vi "Read from Hardware.vi"(8 "error in":errorcluster, 10 "Values in":dbl[](array[numeric]), 11 "Monitor Execution Unit Implementation in":refnum<class "Monitor Execution Unit.lvclass">) -> (0 "error out":errorcluster, 2 "Values out":dbl[](array[numeric]), 3 "Monitor Execution Unit Implementation out":refnum<class "Monitor Execution Unit.lvclass">)   [LabVIEW 2020, in "AIM ARINC 664 Engine.lvlib" / "Implementation.lvlib" / "Monitor Execution Unit.lvclass"]
uses:
  Monitor Execution Unit.lvclass
  Monitor Execution Unit.lvclass/Monitor Execution Unit.ctl
  <instrlib>/AIM GmbH/_AIM 664/AIM664LV.lvlib
  Logging/Frame Logging/Frame Logging.lvlib
  <vilib>/Utility/SystemLogging/NI_SystemLogging.lvlib
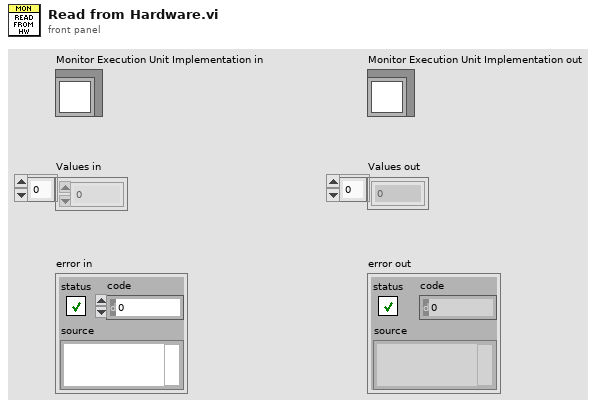
[diagram p1: front panel]
types:
  T1 = typedef "Frame Logging.lvlib/Log_Producer.ctl" = cluster{"Configured":bool, "message queue in":refnum<queue>, "StopNotification":refnum<notifier>}
  T2 = cluster{"QueueStatus":u32, "FramesToRead":u32, "BytesToRead":u32}
  T3 = cluster{"EntryRead":u32, "BytesRead":u32, "Synchronized":u32, "ReadBuffer":u8[]}
  T4 = typedef "Frame.ctl" = cluster{"FwIrigTime":cluster{"TtHigh":u32, "TtLow":u32}, "Payload":u8[], "Lenght":u32}
  T5 = cluster{"TotalByteCount":u32[], "FrameGoodCount":u32[], "FrameErrorCount":u32[], "BytesPerSecond":u32[], "FramesPerSecond":u32[], "PhysErrorCount":u32[], "PreamErrorCount":u32[], "UnaligErrorCount":u32[], "CRCErrorCount":u32[], "IFGErrorCount":u32[], "IPErrorCount":u32[], "MACErrorCount":u32[], "NoSfdErrorCount":u32[], "VLLenErrorCount":u32[], "SNIntegrityErrorCount":u32[], "TrafShapingViolationCount":u32[], "MAC1Short":u32[], "MAC64To127Count":u32[], "MAC128To255Count":u32[], "MAC256To511Count":u32[], "MAC512To1023Count":u32[], "MAC1024To1518Count":u32[], "MACLong":u32[]}
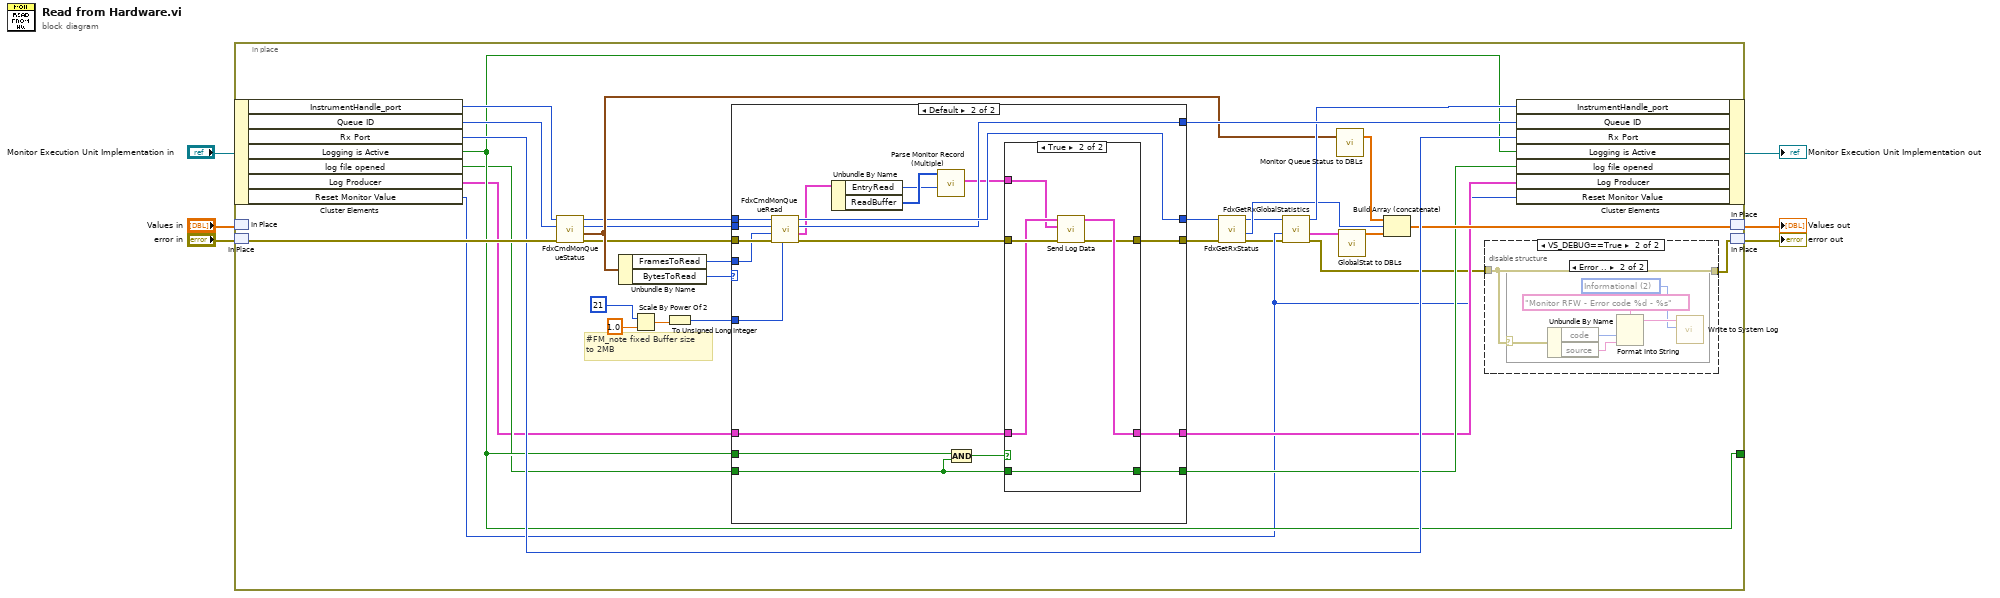
[diagram p0: block diagram]
diagram:
  n1 = in-place {
    in-place-border: [w29] -> _
    # "#FM_note fixed Buffer size\nto 2MB"
    n2 = in-place-cluster #1("Monitor Execution Unit Implementation in") -> ("InstrumentHandle_port"=w38:u32, "Queue ID"=w39:u32, "Rx Port"=w31:u32, "Logging is Active"=w29:bool, "log file opened"=w28:bool, "Log Producer"=w26:T1, "Reset Monitor Value"=w18:u32)
    n3 = in-place-match #2("Values in") -> ()  [unwired: 1 out]
    n4 = in-place-match #3("error in") -> (w37:errorcluster)
    n5 = call <instrlib>:"FdxCmdMonQueueStatus.vi"("error in"=w37, "QueueId"=w39, "InstrumentHandle_port"=w38) -> ("error out"=w24:errorcluster, "QueueStatus"=w32:T2, "QueueIdOut"=w22:u32, "InstrumentHandle_port"=w23:u32)  [unwired: 5 in]
    n6 = Unbundle By Name(w32) -> ("FramesToRead"=w21:u32, "BytesToRead"=w11:u32)
    n7 = Scale By Power Of 2(n=21, x=1.0) -> (x*2^n=w8:dbl)
    n8 = To Unsigned Long Integer(number=w8) -> (unsigned 32bit integer=w7:u32)
    n9 = case shown="Default" w11 {
      tunnel: w24 -> [w42 w61]
      tunnel: w23 -> [w44 w63]
      tunnel: w22 -> [w43 w62]
      tunnel: [w44 w60] -> w34
      tunnel: [w43 w59] -> w35
      tunnel: [w42 w56] -> w36
      tunnel: w21 -> [_ w58]
      tunnel: w29 -> [_ w53]
      tunnel: [w41 w54] -> w27
      tunnel: w28 -> [w41 w51]
      tunnel: w26 -> [w40 w50]
      tunnel: [w40 w49] -> w25
      tunnel: w7 -> [_ w48]
      frame 0 {
      }
      frame Default {
        n10 = call <instrlib>:"FdxCmdMonQueueRead.vi"("MaxReadBytes"=w48, "error in"=w61, "EntryCount"=w58, "QueueId"=w62, "InstrumentHandle_port"=w63) -> ("error out"=w57:errorcluster, "QueueReadOut"=w47:T3, "QueueIdOut"=w59:u32, "InstrumentHandle_port"=w60:u32)  [unwired: 3 in]
        n11 = Unbundle By Name(w47) -> ("EntryRead"=w45:u32, "ReadBuffer"=w46:u8[])
        n12 = call "Parse Monitor Record (Multiple).vi"("record count"=w45, "Record In"=w46) -> ("Payloads"=w55:T4[])  [unwired: 6 in, 3 out]
        n13 = And(x=w53, y=w51) -> (x .and. y?=w52:bool)
        n14 = case shown="True" w52 {
          tunnel: w57 -> [w66 w71]
          tunnel: [w66 w68] -> w56
          tunnel: w55 -> [_ w67]
          tunnel: [w65 w72] -> w54
          tunnel: w51 -> [w65 w72]
          tunnel: w50 -> [w64 w70]
          tunnel: [w64 w69] -> w49
          frame False {
          }
          frame True {
            n15 = call "Send Log Data.vi"("error in"=w71, "Data"=w67, "Log Producer in"=w70) -> ("error out"=w68:errorcluster, "Log Producer out"=w69:T1)  [unwired: 7 in]
          }
        }
      }
    }
    n16 = call <instrlib>:"FdxGetRxStatus.vi"("error in"=w36, "InstrumentHandle_port in"=w34) -> ("error out"=w17:errorcluster, "RxStatus"=w16:u32, "InstrumentHandle_port out"=w15:u32)  [unwired: 6 in, 1 out]
    n17 = call <instrlib>:"FdxGetRxGlobalStatistics.vi"("error in"=w17, "Control"=w18, "InstrumentHandle_port in"=w15) -> ("error out"=w20:errorcluster, "GlobalStat Out"=w14:T5, "InstrumentHandle_port out"=w33:u32)  [unwired: 6 in]
    n18 = call "Monitor Queue Status to DBLs.vi"("MonQueueStatus"=w32) -> ("MonQueueStatusDBLs"=w12:dbl[])  [unwired: 2 in]
    n19 = call "GlobalStat to DBLs.vi"("GlobalStat in"=w14) -> ("GlobalStat DBL Array"=w13:dbl[])  [unwired: 10 in]
    n20 = Build Array (concatenate)(w12, w16, w13) -> (w30:dbl[])
    n21 = disable-structure shown="VS_DEBUG==True" {
      disable-tunnel: w20 -> [w73 w74]
      disable-tunnel: [w73 w74] -> w19
      frame condition #0 (active) {
      }
      frame condition #1 {
        n22 = case shown="Error .." w74 {
          selector: w74 -> [_ w75]
          frame No Error {
          }
          frame Error {
            w78 = 2 items=["Error", "Warning", "Informational"] ("severity")
            n23 = Unbundle By Name(w75) -> ("code"=w77:i32, "source"=w76:string)
            n24 = Format Into String(format string="Monitor RFW - Error code %d - %s", w77, w76) -> (resulting string=w79:string)  [unwired: 2 in, 1 out]
            n25 = call <vilib>:"Write to System Log.vi"("severity"=w78, "message"=w79) -> ()  [unwired: 9 in, 1 out]
          }
        }
      }
    }
    n26 = in-place-cluster #1("InstrumentHandle_port"=w33, "Queue ID"=w35, "Rx Port"=w31, "Logging is Active"=w29, "log file opened"=w27, "Log Producer"=w25, "Reset Monitor Value"=w18) -> (→"Monitor Execution Unit Implementation out":refnum<class "Monitor Execution Unit.lvclass">)
    n27 = in-place-match #2(w30) -> (→"Values out":dbl[])
    n28 = in-place-match #3(w19) -> (→"error out":errorcluster)
  }
